vi "DCS_Trigger_Size_Calculator.vi"(9 "Sample_Rate (Hz)":dbl, 11 "Partical_Velocity (m/s)":dbl) -> (1 "DCS_2_Post_Trigger":dbl, 3 "DCS_1_Pre_Trigger":dbl)   [LabVIEW 2013]
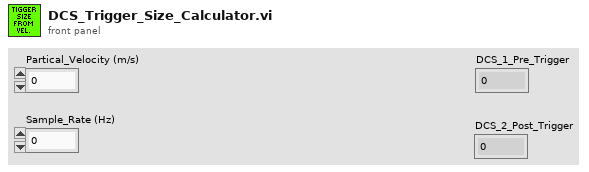
[diagram p1: front panel]
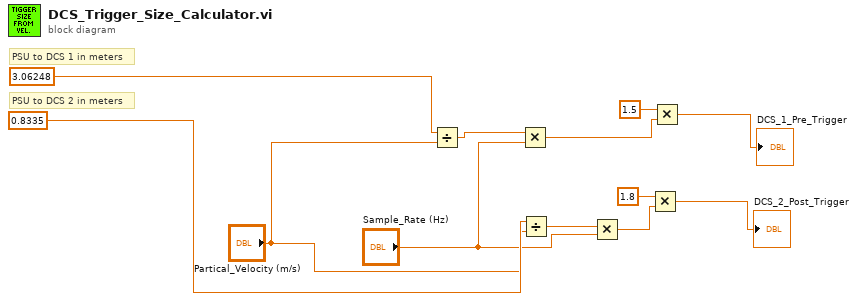
[diagram p0: block diagram]
diagram:
  # "PSU to DCS 1 in meters"
  # "PSU to DCS 2 in meters"
  n1 = Divide(x=3.06248, y="Partical_Velocity (m/s)") -> (x/y=w11:dbl)
  n2 = Multiply(x=w11, y="Sample_Rate (Hz)") -> (x*y=w4:dbl)
  n3 = Divide(x=0.8335, y="Partical_Velocity (m/s)") -> (x/y=w8:dbl)
  n4 = Multiply(x=w8, y="Sample_Rate (Hz)") -> (x*y=w2:dbl)
  n5 = Multiply(x=1.8, y=w2) -> (x*y=→"DCS_2_Post_Trigger":dbl)
  n6 = Multiply(x=1.5, y=w4) -> (x*y=→"DCS_1_Pre_Trigger":dbl)
